vi "TPKT - Read Packet.vi"(8 "error in (no error)":errorcluster, 11 "S7":refnum<class "S7NetCom.lvclass">) -> (0 "error out":errorcluster, 2 "TPDU":T1 format="0x%02x", 3 "S7 out":refnum<class "S7NetCom.lvclass">)   [LabVIEW 2014, in "S7NetCom.lvclass"]
doc: "Reads the TPKT packet from the network and returns the packet data.\n\n_____\nCopyright (c) 2019 Hampel Software Engineering (HSE), released under BSD license. More info can be found on https://dokuwiki.hampel-soft.com/code/hse/s7netcom. Original code published by Marc Christenson, Sisu Devices."
uses:
  S7NetCom.lvclass
  Controls/S7NetCom_HexByteArray.ctl
  Controls/S7NetCom_HexByte.ctl
  S7NetCom.lvclass/S7NetCom.ctl
  TPKT - Validate Header Bytes.vi
  TPKT - Get TDPU Length.vi
  TPKT - Header Bytes 1 and 2--constant.vi
  TPKT - Response Header Mismatch--error.vi
panel:
  # "More info on https://dokuwiki.hampel-soft.com/code/hse/s7netcom\n\nCopyright (c) 2019, HAMPEL SOFTWARE ENGINEERING (HSE)\nOriginal code developed by Marc Christenson, Sisu Devices\nAll rights reserved.\n\nRedistribution and use in source and binary forms, with or without\nmodification, are permitted provided that the following conditions are met:\n\n1. Redistributions of source code must retain the above copyright\n   notice, this list of conditions and the following disclaimer.\n\n2. Redistributions in binary form must reproduce the above copyright\n   notice, this list of conditions and the following disclaimer in the\n   documentation and/or other materials provided with the distribution.\n\n3. All advertising materials mentioning features or use of this software\n   must display the following acknowledgement:\n   This product includes software developed by HAMPEL SOFTWARE ENGINEERING.\n\n4. Neither the name of HAMPEL SOFTWARE ENGINEERING nor the\n   names of its contributors may be used to endorse or promote products\n   derived from this software without specific prior written permission.\n\nTHIS SOFTWARE IS PROVIDED BY HAMPEL SOFTWARE ENGINEERING ''AS IS'' AND ANY\nEXPRESS OR IMPLIED WARRANTIES, INCLUDING, BUT NOT LIMITED TO, THE IMPLIED\nWARRANTIES OF MERCHANTABILITY AND FITNESS FOR A PARTICULAR PURPOSE ARE\nDISCLAIMED. IN NO EVENT SHALL HAMPEL SOFTWARE ENGINEERING BE LIABLE FOR ANY\nDIRECT, INDIRECT, INCIDENTAL, SPECIAL, EXEMPLARY, OR CONSEQUENTIAL DAMAGES\n(INCLUDING, BUT NOT LIMITED TO, PROCUREMENT OF SUBSTITUTE GOODS OR SERVICES;\nLOSS OF USE, DATA, OR PROFITS; OR BUSINESS INTERRUPTION) HOWEVER CAUSED AND\nON ANY THEORY OF LIABILITY, WHETHER IN CONTRACT, STRICT LIABILITY, OR TORT\n(INCLUDING NEGLIGENCE OR OTHERWISE) ARISING IN ANY WAY OUT OF THE USE OF THIS\nSOFTWARE, EVEN IF ADVISED OF THE POSSIBILITY OF SUCH DAMAGE."
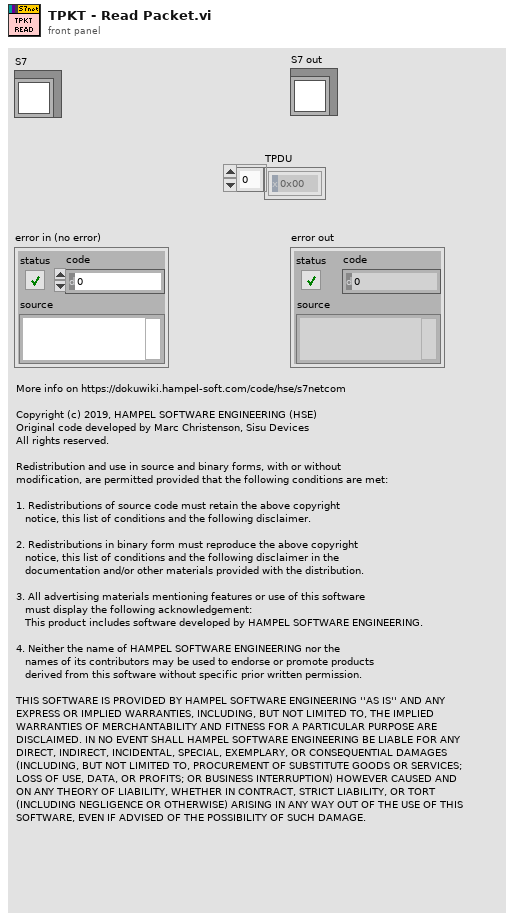
[diagram p1: front panel]
types:
  T1 = typedef "S7NetCom.lvclass/S7NetCom_HexByteArray.ctl" = T2[]
  T2 = typedef "S7NetCom.lvclass/S7NetCom_HexByte.ctl" = u8
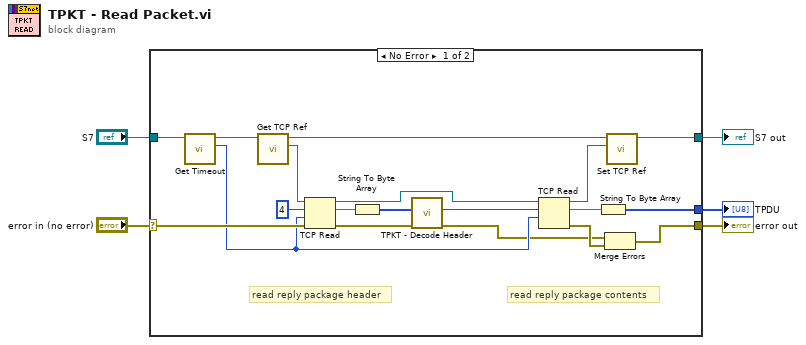
[diagram p0: block diagram]
diagram:
  n1 = case shown="No Error" "error in (no error)" {
    selector: "error in (no error)" -> [w24 w25]
    tunnel: "S7" -> [w23 w26]
    tunnel: [w17 _] -> w3
    tunnel: [w10 w26] -> w2
    tunnel: [w7 w25] -> w1
    frame No Error {
      # "read reply package contents"
      # "read reply package header"
      n2 = call "Get Timeout.vi"("S7NetCom in"=w23) -> ("Timeout [ms]"=w14:i32, "S7NetCom out"=w13:refnum<class "S7NetCom.lvclass">)  [unwired: 9 in]
      n3 = call "Get TCP Ref.vi"("S7NetCom in"=w13) -> ("TCP Ref"=w12:refnum<k5>, "S7NetCom out"=w11:refnum<class "S7NetCom.lvclass">)  [unwired: 9 in]
      n4 = TCP Read(connection ID=w12, bytes to read=4, error in (no error)=w24, 9:w14) -> (connection ID out=w15:refnum<k5>, data out=w21:string, error out=w19:errorcluster)  [unwired: 1 in]
      n5 = String To Byte Array(string=w21) -> (unsigned byte array=w20:u8[])
      n6 = call "TPKT - Decode Header.vi"("error in (no error)"=w19, "TPKT Header"=w20) -> ("error out"=w6:errorcluster, "TPDU Length"=w22:u16)  [unwired: 8 in]
      n7 = TCP Read(connection ID=w15, bytes to read=w22, 9:w14) -> (connection ID out=w9:refnum<k5>, data out=w16:string, error out=w8:errorcluster)  [unwired: 2 in]
      n8 = String To Byte Array(string=w16) -> (unsigned byte array=w17:u8[])
      n9 = Merge Errors(w6, w8) -> (w7:errorcluster)
      n10 = call "Set TCP Ref.vi"("TCP Ref"=w9, "S7NetCom in"=w11) -> ("S7NetCom out"=w10:refnum<class "S7NetCom.lvclass">)  [unwired: 9 in]
    }
    frame Error {
    }
  }
  "S7 out" <- w2
  "error out" <- w1
  "TPDU" <- w3
